vi "Set Multiplexer.vi"(8 "error in":errorcluster, 10 "Multiplexer":cluster{"Index":u16, "Sub-Index":u8} {"Sub-Index" format="%02x"; "Index" format="%04x"}, 11 "SDO Transfer in":refnum<class "SDO Transfer.lvclass">) -> (0 "error out":errorcluster, 3 "SDO Transfer out":refnum<class "SDO Transfer.lvclass">)   [LabVIEW 2020, in "SDO Manager.lvlib" / "SDO Transfer.lvclass"]
uses:
  SDO Transfer.lvclass
  SDO Transfer.lvclass/SDO Transfer.ctl
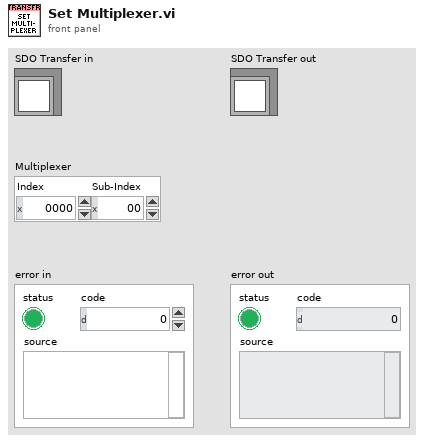
[diagram p1: front panel]
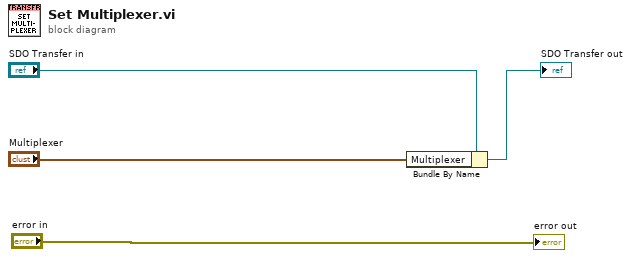
[diagram p0: block diagram]
diagram:
  n1 = Bundle By Name(cluster="SDO Transfer in", "Multiplexer"="Multiplexer") -> (→"SDO Transfer out":refnum<class "SDO Transfer.lvclass">)
  "error out" <- "error in"
